vi "Check Previous Values.vi"(11 "values":dbl[](array[numeric])) -> (1 "values modified?":bool, 2 "modified indices":i32[](array[numeric]), 3 "values out":dbl[](array[numeric]))   [LabVIEW 2020, in "Ballard ARINC 429 Engine.lvlib" / "Implementation.lvlib" / "Tx Scheduled Labels Execution Unit.lvclass"]
uses:
  Tx Scheduled Labels Execution Unit.lvclass
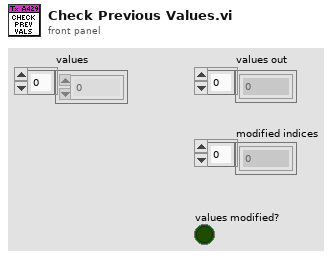
[diagram p1: front panel]
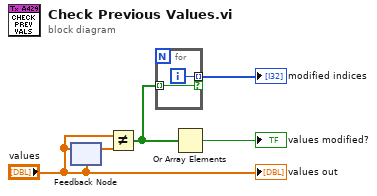
[diagram p0: block diagram]
diagram:
  n1 = feedback #1("values") -> (w5:dbl[])
  n2 = feedback-in #1("values") -> ()
  n3 = Not Equal?(x="values", y=w5) -> (x != y?=w4:bool[])
  n4 = for {
    tunnel: w4 -> [w6] mode=indexing
    tunnel: [w7] -> w2 mode=indexing if=w6
    i -> [w7]
  }
  "modified indices" <- w2
  n5 = Or Array Elements(Boolean array=w4) -> (logical OR=→"values modified?":bool)
  "values out" <- "values"
